vi "PathPlanner_PathFinder_GetWorkerDebug.vi"() -> (3 "PathFinderWorkerDebug":T3 {"CurrentPath"."Y" format="%14.3f"; "CurrentPath"."X" format="%14.3f"; "ExtractedFieldPosPath"."Y" step=0.25 format="%14.3f"; "ExtractedFieldPosPath"."X" format="%14.3f"})   [LabVIEW 2019, in "PathPlanner24.lvlib"]
doc: "Get debug information for Path Finder worker"
uses:
  PathPlanner24.lvlib
  TypeDef/PathPlannerFinderGridPosition.ctl
  <vilib>/Rock Robotics/WPI/ThirdParty/JAS_Junk/TrajLib/TypeDef/TRANSLATION2D.ctl
  <vilib>/robotics/Navigation/shared/WorldMap/OccupancyGridWorldMap/NI_Robotics_OccupancyGridWorldMap.lvclass
  <vilib>/robotics/Navigation/shared/MapNode/AbstractDstarNode/NI_Robotics_AbstractDstarNode.lvclass
  PathPlanner_PathFinder_Globals.vi
  <vilib>/Rock Robotics/WPI/ThirdParty/JAS_Junk/TrajLib/Trajectory_Library.lvlib
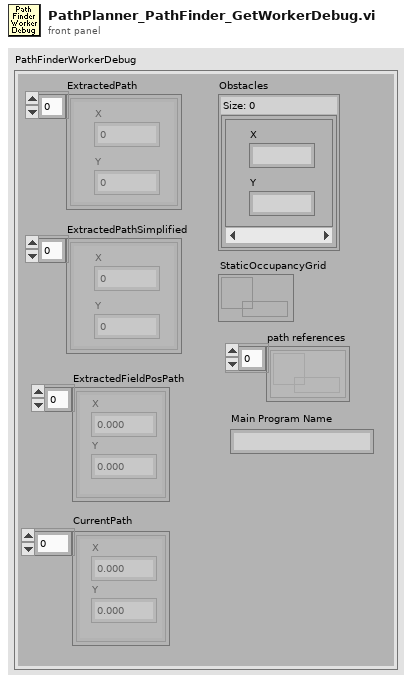
[diagram p1: front panel]
types:
  T1 = typedef "PathPlanner24.lvlib/PathPlannerFinderGridPosition.ctl" = cluster{"X":i32, "Y":i32}
  T2 = typedef "Trajectory_Library.lvlib/TRANSLATION2D.ctl" = cluster{"X":dbl, "Y":dbl}
  T3 = cluster{"ExtractedPath":T1[], "ExtractedPathSimplified":T1[], "ExtractedFieldPosPath":T2[], "CurrentPath":T2[], "Obstacles":set{T1}, "StaticOccupancyGrid":refnum<data-value>, "path references":refnum<data-value>[], "Main Program Name":string}
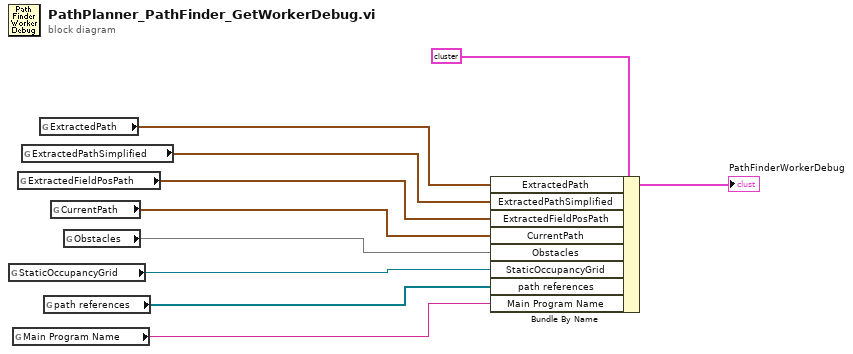
[diagram p0: block diagram]
diagram:
  n1 = global read "PathPlanner_PathFinder_Globals.vi" "StaticOccupancyGrid"() -> (w3:refnum<data-value>)
  n2 = global read "PathPlanner_PathFinder_Globals.vi" "Main Program Name"() -> (w1:string)
  n3 = global read "PathPlanner_PathFinder_Globals.vi" "ExtractedFieldPosPath"() -> (w6:T2[])
  n4 = global read "PathPlanner_PathFinder_Globals.vi" "ExtractedPathSimplified"() -> (w7:T1[])
  n5 = global read "PathPlanner_PathFinder_Globals.vi" "ExtractedPath"() -> (w8:T1[])
  n6 = global read "PathPlanner_PathFinder_Globals.vi" "path references"() -> (w2:refnum<data-value>[])
  n7 = global read "PathPlanner_PathFinder_Globals.vi" "CurrentPath"() -> (w5:T2[])
  n8 = global read "PathPlanner_PathFinder_Globals.vi" "Obstacles"() -> (w4:set{T1})
  n9 = Bundle By Name(cluster=T3 {"ExtractedPath"=[], "ExtractedPathSimplified"=[], "ExtractedFieldPosPath"=[], "CurrentPath"=[], "Obstacles"={}, "StaticOccupancyGrid"=refnum, "path references"=[], "Main Program Name"=""} ("PathFinderWorkerDebug"), "ExtractedPath"=w8, "ExtractedPathSimplified"=w7, "ExtractedFieldPosPath"=w6, "CurrentPath"=w5, "Obstacles"=w4, "StaticOccupancyGrid"=w3, "path references"=w2, "Main Program Name"=w1) -> (→"PathFinderWorkerDebug":T3)
